vi "assignment1.vi"() -> ()   [LabVIEW 2023]
uses:
  <vilib>/Utility/error.llb/Trim Whitespace One-Sided.vi
  <vilib>/Utility/file.llb/Write Delimited Spreadsheet (string).vi
panel:
  out "error out":errorcluster
  in  "delimiter (\\t)":string="\t"
  in  "format (%s)":string="%s"
  in  "file path (dialog if empty)":path
  in  "stop":bool
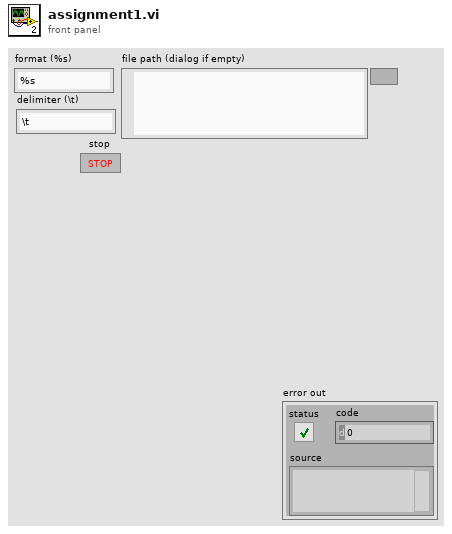
[diagram p1: front panel]
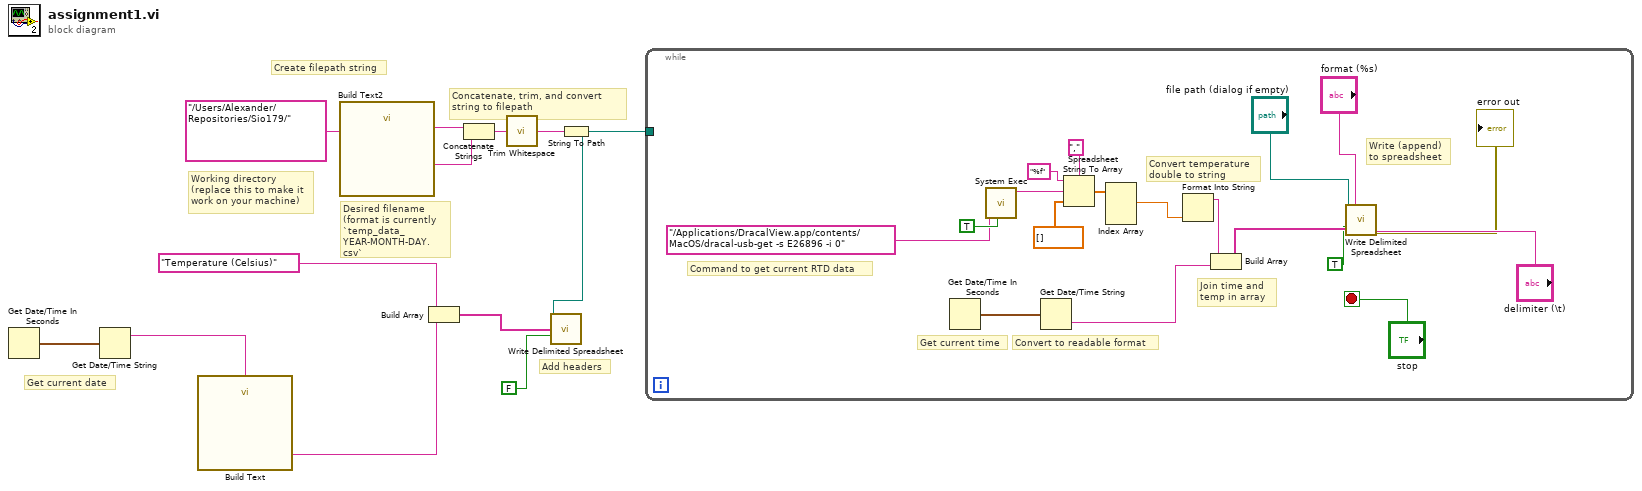
[diagram p0: block diagram]
diagram:
  # "Add headers"
  # "Get current date"
  # "Concatenate, trim, and convert string to filepath"
  # "Desired filename (format is currently `temp_data_YEAR-MONTH-DAY.csv`"
  # "Working directory (replace this to make it work on your machine)"
  # "Create filepath string"
  n1 = Get Date/Time In Seconds() -> (seconds since 1Jan1904=w8:timestamp)
  n2 = Get Date/Time String(seconds (now)=w8) -> (date string=w2:string)  [unwired: 2 in, 1 out]
  n3 = call "Build Text"("date"=w2) -> ("Result"=w6:string)  [unwired: 13 in, 1 out]
  n4 = call "Build Text2"() -> ("Result"=w1:string)  [unwired: 14 in, 1 out]
  n5 = Build Array("Temperature (Celsius)", w6) -> (w5:string[])
  n6 = Concatenate Strings("/Users/Alexander/Repositories/Sio179/", w1) -> (w9:string)
  n7 = call <vilib>:"Trim Whitespace.vi"("string"=w9) -> ("trimmed string"=w11:string)  [unwired: 1 in]
  n8 = String To Path(string=w11) -> (path=w3:path)
  n9 = call-poly <vilib>:"Write Delimited Spreadsheet.vi"("file path (dialog if empty)"=w3, "1D data"=w5, "append to file? (new file:F)"=FALSE) -> ()  [unwired: 11 in, 2 out]
  n10 = while {
    tunnel: w3 -> [_]
    stop <- "stop" stop-if-true
    # "Command to get current RTD data"
    # "Join time and temp in array"
    # "Convert temperature double to string"
    # "Convert to readable format"
    # "Get current time"
    # "Write (append) to spreadsheet"
    n11 = Get Date/Time In Seconds() -> (seconds since 1Jan1904=w18:timestamp)
    n12 = call <vilib>:"System Exec.vi"("run minimized? (F)"=TRUE, "command line"="/Applications/DracalView.app/contents/MacOS/dracal-usb-get -s E26896 -i 0") -> ("standard output"=w24:string)  [unwired: 6 in, 3 out]
    n13 = Get Date/Time String(seconds (now)=w18) -> (time string=w22:string)  [unwired: 2 in, 1 out]
    n14 = Spreadsheet String To Array(delimiter (Tab)=",", format string="%f", spreadsheet string=w24, array type (2D Dbl)=dbl[] [] ("Array")) -> (array=w27:dbl[])
    n15 = Index Array(array=w27) -> (element #1=w21:dbl)  [unwired: 3 in, 2 out]
    n16 = Format Into String(w21) -> (resulting string=w20:string)  [unwired: 3 in, 1 out]
    n17 = Build Array(w20, w22) -> (w19:string[])
    n18 = call-poly <vilib>:"Write Delimited Spreadsheet.vi"("file path (dialog if empty)"="file path (dialog if empty)", "format (%s)"="format (%s)", "1D data"=w19, "append to file? (new file:F)"=TRUE, "delimiter (\\t)"="delimiter (\\t)") -> ("error out"=→"error out":errorcluster)  [unwired: 9 in, 1 out]
  }
